vi "Pre_Loop_Initialization_FGV.vi"(8 "error in (no error)":errorcluster, 10 "DUT":string, 11 "VI in":refnum<vi>) -> (0 "error out":errorcluster, 2 "queue out":refnum<queue>, 3 "User Event out":refnum<user-event>)   [LabVIEW 2024, in "MCU_Flashing.lvlib"]
doc: "This VI\n------------------------------------------------\nPer_Loop_Initialize\n------------------------------------------------\n-Generate the Communication Queue Reference with FGV.\n-Get the Common User Events Reference at Application Level."
uses:
  MCU_Flashing.lvlib
  UserEvents/Controls/User_Events_Action_Control.ctl
  PrivateControls/FGV_Queue_Control.ctl
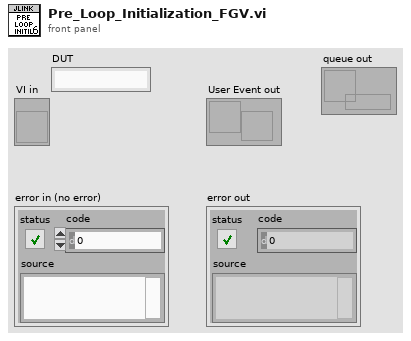
[diagram p1: front panel]
types:
  T1 = typedef "MCU_Flashing.lvlib/User_Events_Action_Control.ctl" = enum16{"Get", "Create", "Destroy"}
  T2 = cluster{"Message":string, "Message Data":variant}
  T3 = typedef "MCU_Flashing.lvlib/FGV_Queue_Control.ctl" = enum16{"Release", "Get", "Set"}
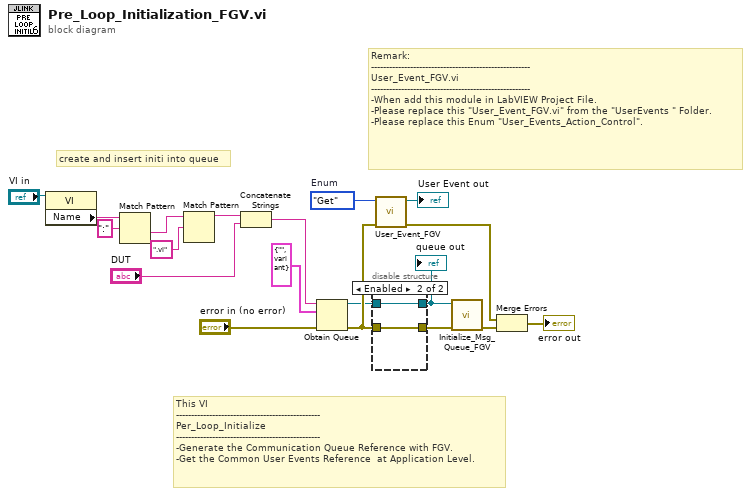
[diagram p0: block diagram]
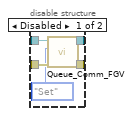
[diagram p2: hidden frame]
diagram:
  w14 = User_Events_Action_Control."Get"  # Enum
  # "Remark:\n-----------------------------------------------------\nUser_Event_FGV.vi\n-----------------------------------------------------\n-When add this module in LabVIEW Project File.\n-Please replace this \"User_Event_FGV.vi\" from the \"UserEvents \" Folder.\n-Please replace this Enum \"User_Events_Action_Control\"."
  # "This VI\n------------------------------------------------\nPer_Loop_Initialize\n------------------------------------------------\n-Generate the Communication Queue Reference with FGV.\n-Get the Common User Events Reference  at Application Level."
  # "create and insert initi into queue"
  n1 = property class="VI"(reference="VI in") -> ("Name"=w7:string)  [unwired: 1 in, 2 out]
  n2 = Match Pattern(string=w7, regular expression=":") -> (after substring=w5:string)  [unwired: 1 in, 3 out]
  n3 = Match Pattern(string=w5, regular expression=".vi") -> (before substring=w3:string)  [unwired: 1 in, 3 out]
  n4 = Concatenate Strings(w3, "DUT") -> (w2:string)
  n5 = Obtain Queue(name (unnamed)=w2, element data type=T2 {"Message"="", "Message Data"=variant} ("Message Cluster"), error in (no error)="error in (no error)") -> (queue out=w13:refnum<queue>, error out=w15:errorcluster)  [unwired: 2 in, 1 out]
  n6 = disable-structure shown="Enabled" {
    disable-tunnel: w15 -> [w23 w25]
    disable-tunnel: w13 -> [w22 w24]
    disable-tunnel: [w21 w25] -> w11
    disable-tunnel: [_ w24] -> w8
    frame Disabled {
      n7 = call "Queue_Comm_FGV.vi"("error in (no error)"=w23, "Enum"=FGV_Queue_Control."Set", "queue in"=w22) -> ("error Out"=w21:errorcluster)  [unwired: 7 in, 1 out]
    }
    frame Enabled {
    }
  }
  "queue out" <- w8
  n8 = call "User_Event_FGV.vi"("error in (no error)"=w15, "Enum"=w14) -> ("error out"=w17:errorcluster, "User Event out"=→"User Event out":refnum<user-event>)  [unwired: 8 in]
  n9 = call "Initialize_Msg_Queue_FGV.vi"("error in (no error)"=w11, "queue in"=w8) -> ("error out"=w18:errorcluster)  [unwired: 9 in]
  n10 = Merge Errors(w17, w18) -> (→"error out":errorcluster)
